vi "test2.vi"() -> ()   [LabVIEW 2021]
uses:
  IFurniture/IFurniture.lvclass
panel:
  out "price":dbl
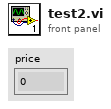
[diagram p1: front panel]
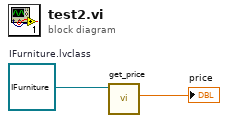
[diagram p0: block diagram]
diagram:
  w2 = refnum<class "IFurniture.lvclass"> refnum  # IFurniture.lvclass
  n1 = call-dynamic "get_price.vi"("IFurniture in"=w2) -> ("price"=→"price":dbl)  [unwired: 8 in, 2 out]
